vi "wavelength scan.vi"() -> ()   [LabVIEW 2012]
panel:
  out "XY Graph":cluster{"Y":dbl[], "Y":dbl[]}[](graph)
  in  "Online":bool
  out "Power2 (W)":dbl(graph)=-5.33e-06
  out "Power1 (W)":dbl format="%.3p"
  in  "Wait (mS)":u32=1000
  out "OphirPM":T1={"Ophir-Ref"=refnum, "Ophir-Device"=1000, "Ophir-Channel"=0}
  out "Waveform Chart":dbl(graph)
  in  "Lambda Step (nm)":dbl=5e-05 format="%.5f"
  in  "Lambda Stop (nm)":dbl=828.299 format="%.5f"
  in  "Lambda Start (nm)":dbl=828.297 format="%.5f"
  in  "step_size":dbl=0.00025 format="%#_6p"
  in  "Device In":refnum<visa-resource-name>="Pro8000"
  in  "Settings":T2={"Module"=enum."Off Line TEC", "OnLineTEC"=23.261520000000402, "OnLineLD"=0.1722, "OffLineTEC"=29.56374999999997, "OffLineLD"=0.173, "EtalonTEC"=26.4, "TSOA-TEC"=18.0} {"OffLineLD" min=0.0 max=0.175 step=0.001 format="%.3p"; "OnLineLD" min=0.0 max=0.175 step=0.001 format="%.3p"; "TSOA-TEC" format="%.2g"; "EtalonTEC" format="%.2g"; "OffLineTEC" min=0.0 max=30.0 step=0.1 format="%.3g"; "OnLineTEC" min=0.0 max=30.0 step=0.1 format="%.3g"}
  out "Readings":T3={"OnLineTEC"=23.2759037, "OnLineLD"=0.172207043, "OffLineTEC"=29.5800114, "OffLineLD"=0.17301172, "EtalonTEC"=-12.375, "TSOA-TEC"=18.9921513, "Pro8000"=TRUE, "OnLine TEC"=TRUE, "OnLine LD"=TRUE, "OffLine TEC"=TRUE, "OffLine LD"=TRUE, "Etalon TEC"=FALSE, "TSOA TEC"=TRUE} {"OffLineLD" format="%.4g"; "OnLineLD" format="%.4g"; "TSOA-TEC" format="%.3g"; "EtalonTEC" format="%.3g"; "OffLineTEC" format="%.3g"; "OnLineTEC" format="%.3g"}
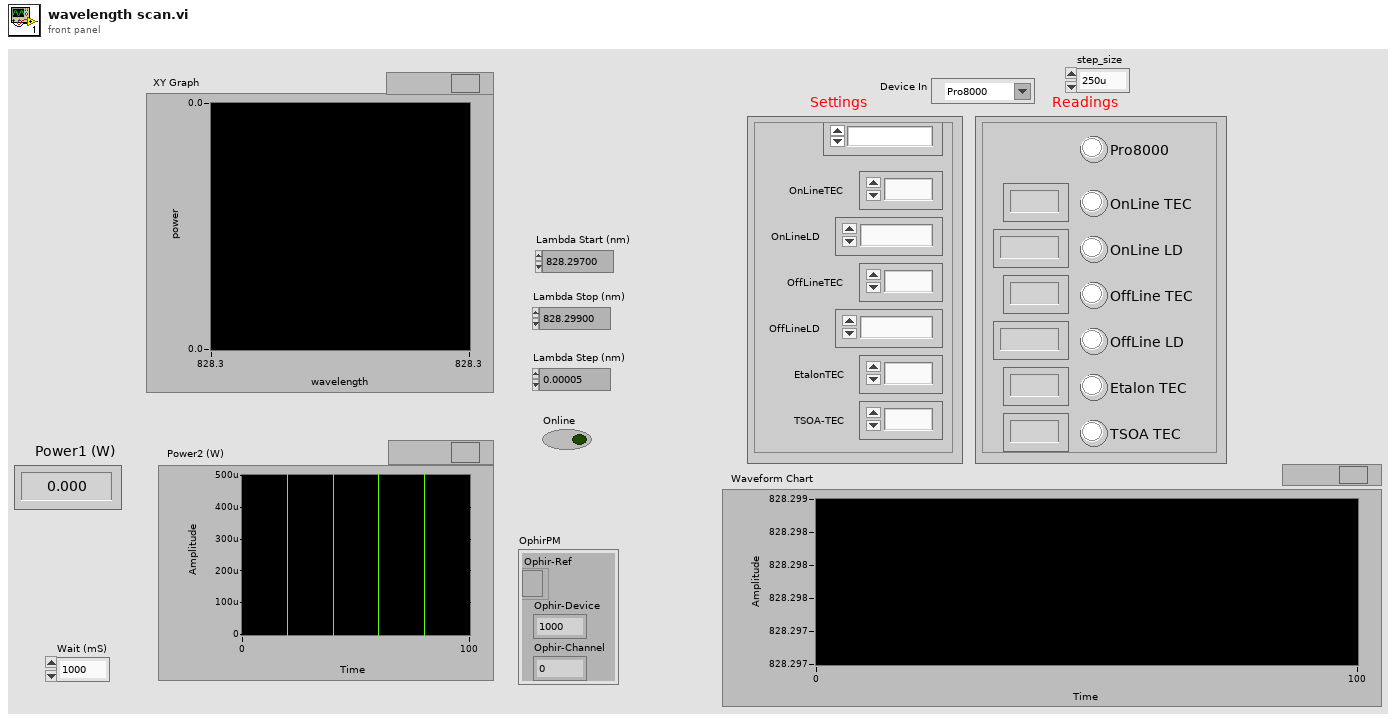
[diagram p1: front panel]
types:
  T1 = cluster{"Ophir-Ref":refnum<k7>, "Ophir-Device":i32, "Ophir-Channel":i32}
  T2 = cluster{"Module":enum16{"On Line TEC", "On Line LD", "Off Line TEC", "Off Line LD", "Etalon TEC", "TSOA TEC"}, "OnLineTEC":dbl, "OnLineLD":dbl, "OffLineTEC":dbl, "OffLineLD":dbl, "EtalonTEC":dbl, "TSOA-TEC":dbl}
  T3 = cluster{"OnLineTEC":dbl, "OnLineLD":dbl, "OffLineTEC":dbl, "OffLineLD":dbl, "EtalonTEC":dbl, "TSOA-TEC":dbl, "Pro8000":bool, "OnLine TEC":bool, "OnLine LD":bool, "OffLine TEC":bool, "OffLine LD":bool, "Etalon TEC":bool, "TSOA TEC":bool}
  T4 = enum16{"Open_TL", "Close_TL", "Verify_ID", "TEC_Sensor", "SET", "READ", "ON", "OFF", "Set_Limits", "Read_Limits", "Enable_Status", "Read_Status"}
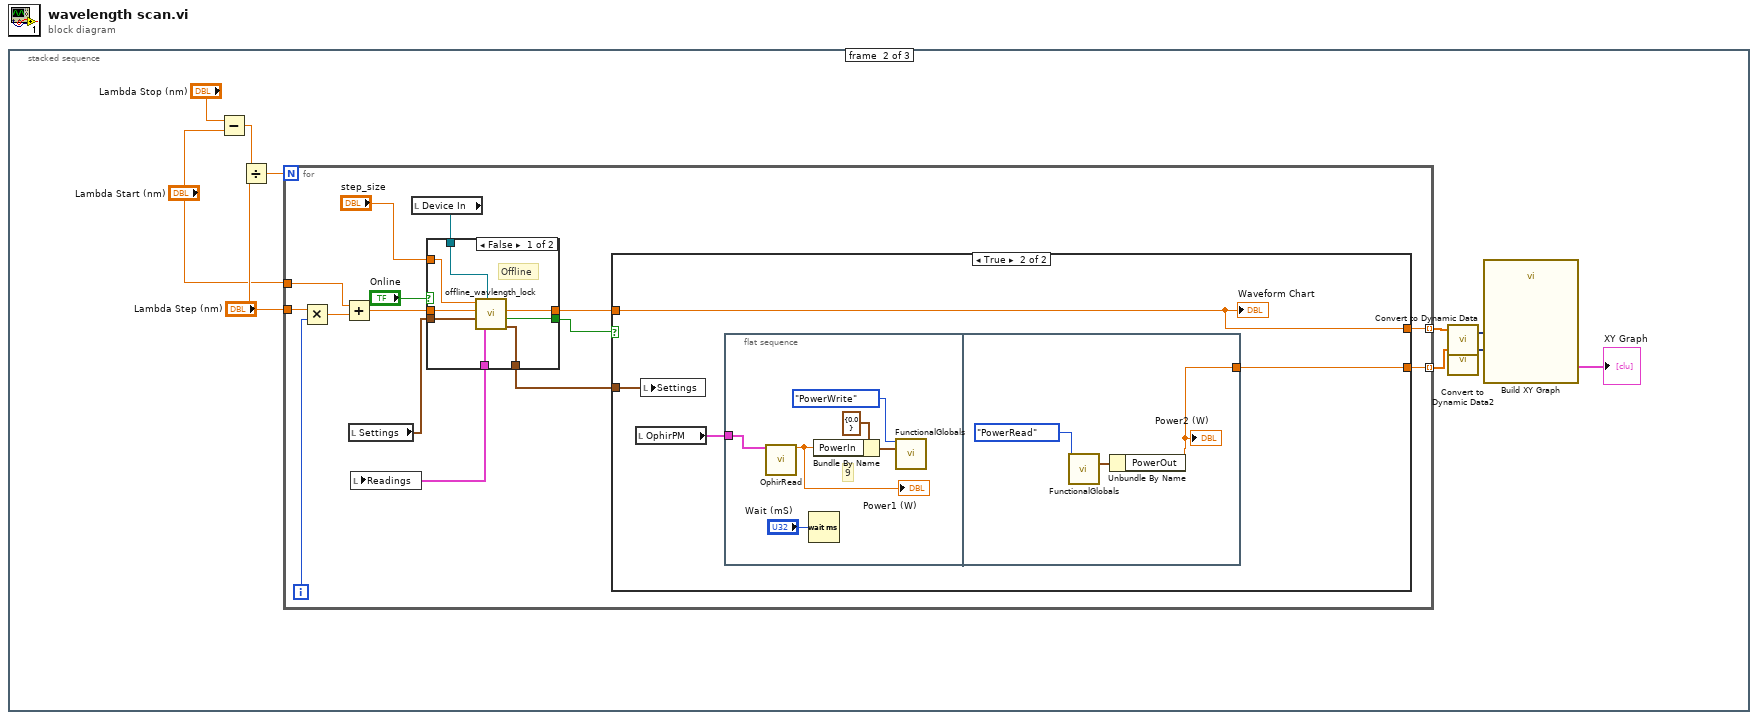
[diagram p0: block diagram]
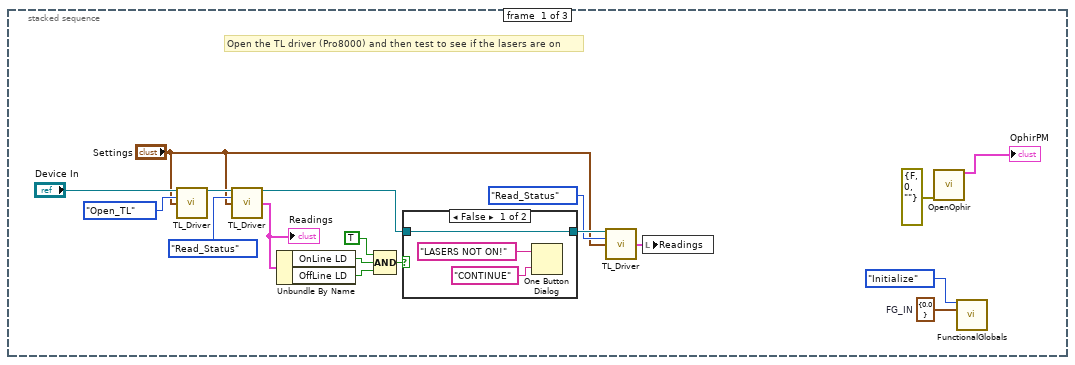
[diagram p2: hidden frame]
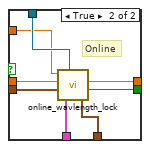
[diagram p4: hidden frame]
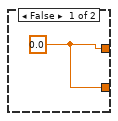
[diagram p5: hidden frame]
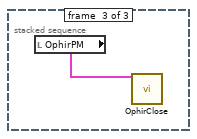
[diagram p6: hidden frame]
diagram:
  n1 = stacked-sequence {
    frame #0 {
      w2 = cluster{"PowerIn":dbl} {"PowerIn"=0.0}  # FG_IN
      # "Open the TL driver (Pro8000) and then test to see if the lasers are on"
      n2 = call "TL_Driver.vi"("Device In"="Device In", "Commands"=T4."Open_TL", "Settings"="Settings") -> ("Device Out"=w7:refnum<visa-resource-name>)  [unwired: 9 in, 3 out]
      n3 = call "TL_Driver.vi"("Device In"=w7, "Commands"=T4."Read_Status", "Settings"="Settings") -> ("Device Out"=w10:refnum<visa-resource-name>, "Readings"=w9:T3)  [unwired: 9 in, 2 out]
      "Readings" <- w9
      n4 = Unbundle By Name(w9) -> ("OnLine LD"=w15:bool, "OffLine LD"=w14:bool)
      n5 = Compound Arithmetic op=AND(TRUE, w15, w14) -> (w16:bool)
      n6 = case shown="False" w16 {
        tunnel: w10 -> [w19 w22]
        tunnel: [w19 w22] -> w12
        frame False {
          n7 = One Button Dialog(message="LASERS NOT ON!", button name ("OK")="CONTINUE") -> ()  [unwired: 1 out]
        }
        frame True {
        }
      }
      n8 = call "TL_Driver.vi"("Device In"=w12, "Commands"=T4."Read_Status", "Settings"="Settings") -> ("Readings"=w17:T3)  [unwired: 9 in, 3 out]
      n9 = local write "Readings"(w17) -> ()
      n10 = call "OpenOphir.vi"("error in (no error)"=errorcluster {"status"=FALSE, "code"=0, "source"=""}) -> ("OphirPM"=→"OphirPM":T1)  [unwired: 13 in, 1 out]
      n11 = call "FunctionalGlobals.vi"("FG_Control"=enum16{"Initialize", "PowerRead", "PowerWrite"}."Initialize", "FG_IN"=w2) -> ()  [unwired: 13 in, 1 out]
    }
    frame #1 {
      n12 = Subtract(x="Lambda Stop (nm)", y="Lambda Start (nm)") -> (x-y=w32:dbl)
      n13 = Divide(x=w32, y="Lambda Step (nm)") -> (x/y=w31:dbl)
      n14 = for {
        N: w31 -> [_]
        tunnel: "Lambda Step (nm)" -> [w46]
        tunnel: "Lambda Start (nm)" -> [w45]
        tunnel: [w34] -> w26 mode=indexing
        tunnel: [w33] -> w24 mode=indexing
        i -> [w47]
        n15 = Multiply(x=w46, y=w47) -> (x*y=w44:dbl)
        n16 = Add(x=w45, y=w44) -> (x+y=w43:dbl)
        n17 = local read "Settings"() -> (w41:T2)
        n18 = local read "Device In"() -> (w42:refnum<visa-resource-name>)
        n19 = case shown="False" "Online" {
          tunnel: w43 -> [w53 w63]
          tunnel: w42 -> [w54 w62]
          tunnel: w41 -> [w52 w61]
          tunnel: [w51 w60] -> w40
          tunnel: [w49 w59] -> w36
          tunnel: [w48 w58] -> w39
          tunnel: [w50 w57] -> w38
          tunnel: "step_size" -> [w55 w56]
          frame False {
            # "Offline"
            n20 = call "offline_wavlength_lock.vi"("Device"=w54, "Settings In"=w52, "Lambda Off Set (nm)"=w53, "step_size"=w55) -> ("Settings Out"=w50:T2, "Wavelength Lock Offline"=w49:bool, "Lambda Off Read (nm)"=w48:dbl, "Readings"=w51:T3)  [unwired: 1 in]
          }
          frame True {
            # "Online"
            n21 = call "online_wavlength_lock.vi"("Device"=w62, "Settings In"=w61, "Lambda On Set (nm)"=w63, "step_size"=w56) -> ("Settings Out"=w57:T2, "Wavelength Lock Online"=w59:bool, "Lambda On Read (nm)"=w58:dbl, "Readings"=w60:T3)  [unwired: 1 in]
          }
        }
        n22 = local write "Readings"(w40) -> ()
        n23 = case shown="True" w36 {
          tunnel: w39 -> [_ w66]
          tunnel: w38 -> [_ w68]
          tunnel: [w64 w66] -> w34
          tunnel: [w64 w65] -> w33
          frame False {
            w64 = 0.0
          }
          frame True {
            n24 = local read "OphirPM"() -> (w67:T1)
            n25 = local write "Settings"(w68) -> ()
            n26 = flat-sequence {
              tunnel: w67 -> [w70]
              tunnel: [w75] -> w65
              frame #0 {
                # "9"
                n27 = call "OphirRead.vi"("OphirPM"=w70) -> ("Power (W)"=w69:dbl)  [unwired: 12 in, 2 out]
                "Power1 (W)" <- w69
                n28 = Wait (ms)(milliseconds to wait="Wait (mS)") -> ()  [unwired: 1 out]
                n29 = Bundle By Name(cluster=cluster{"PowerIn":dbl} {"PowerIn"=0.0} ("FG_IN"), "PowerIn"=w69) -> (w72:cluster{"PowerIn":dbl})
                n30 = call "FunctionalGlobals.vi"("FG_Control"=enum16{"Initialize", "PowerRead", "PowerWrite"}."PowerWrite", "FG_IN"=w72) -> ()  [unwired: 13 in, 1 out]
              }
              frame #1 {
                n31 = call "FunctionalGlobals.vi"("FG_Control"=enum16{"Initialize", "PowerRead", "PowerWrite"}."PowerRead") -> ("FG_OUT"=w76:cluster{"PowerOut":dbl})  [unwired: 14 in]
                n32 = Unbundle By Name(w76) -> ("PowerOut"=w75:dbl)
                "Power2 (W)" <- w75
              }
            }
            "Waveform Chart" <- w66
          }
        }
      }
      n33 = call "Convert to Dynamic Data"("Array"=w26) -> ("Dynamic Data Type"=w25:dynamicdata)  [unwired: 3 in]
      n34 = call "Convert to Dynamic Data2"("Array"=w24) -> ("Dynamic Data Type"=w23:dynamicdata)  [unwired: 3 in]
      n35 = call "Build XY Graph"("Y Input"=w23, "X Input"=w25) -> ("XY Graph"=→"XY Graph":cluster{"Y":dbl[], "Y":dbl[]}[])  [unwired: 3 in, 6 out]
    }
    frame #2 {
      n36 = local read "OphirPM"() -> (w78:T1)
      n37 = call "OphirClose.vi"("OphirPM"=w78) -> ()  [unwired: 18 in, 1 out]
    }
  }
